vi "Database Connection Manager.vi"(6 "Return Data (T)":bool=TRUE, 7 "ConnectionString":string, 8 "error in (no error)":errorcluster, 9 "Command Text":string, 10 "Method":T1, 11 "ADODB._Connection In":refnum<k7>) -> (0 "error out":errorcluster, 1 "Rows Fetched":i32, 2 "Data":string[][](array[string]), 3 "ADODB._Connection Out":refnum<k7>)   [LabVIEW 2015]
uses:
  Ctl/database_Method.ctl
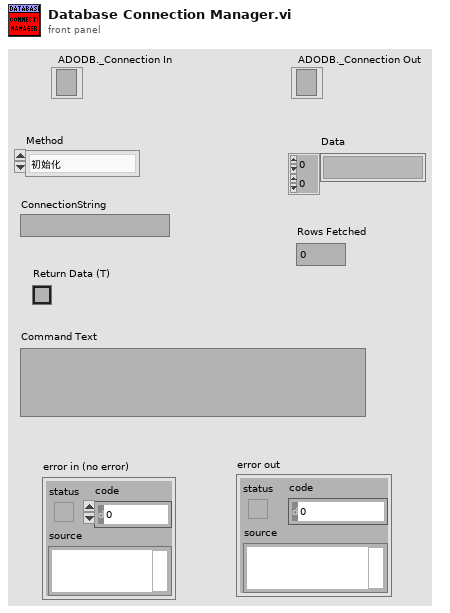
[diagram p1: front panel]
types:
  T1 = typedef "database_Method.ctl" = enum16{"初始化", "查询", "关闭"}
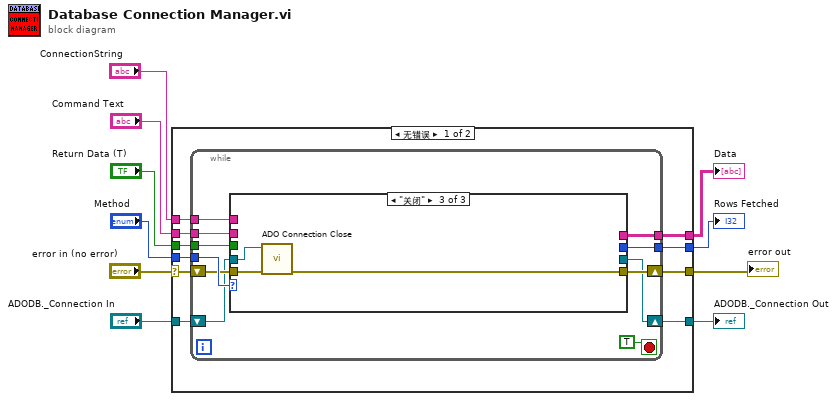
[diagram p0: block diagram]
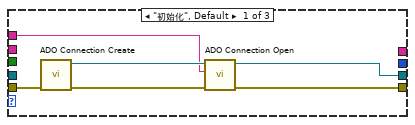
[diagram p2: hidden frame]
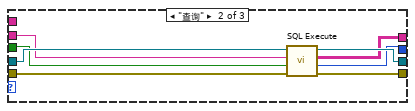
[diagram p3: hidden frame]
diagram:
  n1 = case shown="无错误" "error in (no error)" {
    selector: "error in (no error)" -> [w19 w49]
    tunnel: "Method" -> [w20 _]
    tunnel: "ConnectionString" -> [w18 _]
    tunnel: "Return Data (T)" -> [w17 _]
    tunnel: "Command Text" -> [w16 _]
    tunnel: [w15 _] -> w5
    tunnel: [w14 _] -> w4
    tunnel: [w13 w49] -> w3
    tunnel: "ADODB._Connection In" -> [w12 _]
    tunnel: [w11 _] -> w1
    frame No Error {
      n2 = while {
        tunnel: w20 -> [w31]
        shift-right: [w28] -> w13
        shift-left: w19 -> [w29]
        shift-right: [w27] -> w11
        shift-left: w12 -> [w25]
        tunnel: w18 -> [w26]
        tunnel: w17 -> [w24]
        tunnel: w16 -> [w23]
        tunnel: [w22] -> w15
        tunnel: [w21] -> w14
        stop <- TRUE stop-if-true
        n3 = case shown="\"关闭\"" w31 {
          tunnel: w29 -> [w37 w45 w47]
          tunnel: [w34 w42 w46] -> w28
          tunnel: [w33 w43 _] -> w27
          tunnel: w26 -> [w32 _ _]
          tunnel: w25 -> [_ w44 w48]
          tunnel: w24 -> [_ w41 _]
          tunnel: w23 -> [_ w40 _]
          tunnel: [_ w39 _] -> w22
          tunnel: [_ w38 _] -> w21
          frame "初始化", Default {
            n4 = call "ADO Connection Create.vi"("error in (no error)"=w37) -> ("error out"=w36:errorcluster, "ADODB._Connection Out"=w35:refnum<k7>)  [unwired: 9 in]
            n5 = call "ADO Connection Open.vi"("error in (no error)"=w36, "ConnectionString"=w32, "ADODB._Connection In"=w35) -> ("error out"=w34:errorcluster, "ADODB._Connection Out"=w33:refnum<k7>)  [unwired: 7 in]
          }
          frame "查询" {
            n6 = call "SQL Execute.vi"("error in (no error)"=w45, "Return Data (T)"=w41, "Command Text"=w40, "ADODB._Connection In"=w44) -> ("error out"=w42:errorcluster, "Rows Fetched"=w38:i32, "Data"=w39:string[][], "ADODB._Connection Out"=w43:refnum<k7>)  [unwired: 4 in]
          }
          frame "关闭" {
            n7 = call "ADO Connection Close.vi"("error in (no error)"=w47, "ADODB._Connection In"=w48) -> ("error out"=w46:errorcluster)  [unwired: 8 in, 1 out]
          }
        }
      }
    }
    frame Error {
    }
  }
  "Data" <- w5
  "Rows Fetched" <- w4
  "ADODB._Connection Out" <- w1
  "error out" <- w3
